vi "Initiaize.vi"(8 "error in (no error)":errorcluster, 11 "Pcal GUI in":refnum<class "Pcal GUI.lvclass">) -> (0 "error out":errorcluster, 3 "Pcal GUI out":refnum<class "Pcal GUI.lvclass">)   [LabVIEW 2015, in "Pcal GUI.lvclass"]
uses:
  Pcal GUI.lvclass
  Pcal GUI.lvclass/Pcal GUI.ctl
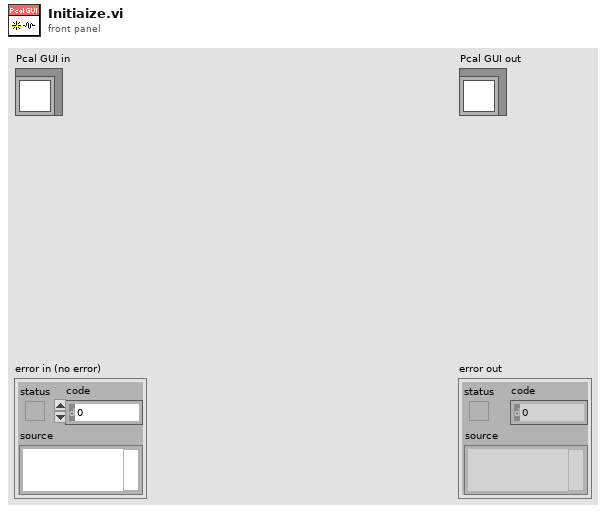
[diagram p1: front panel]
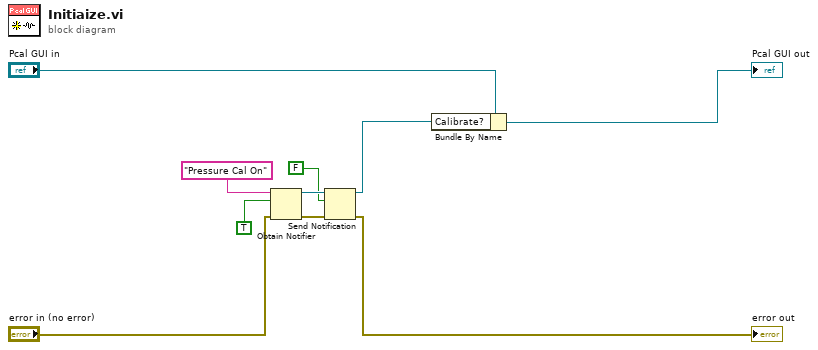
[diagram p0: block diagram]
diagram:
  n1 = Obtain Notifier(name (unnamed)="Pressure Cal On", notification data type=TRUE, error in (no error)="error in (no error)") -> (notifier out=w6:refnum<notifier>, error out=w4:errorcluster)  [unwired: 1 in, 1 out]
  n2 = Send Notification(notification=FALSE, notifier=w6, error in (no error)=w4) -> (notifier out=w3:refnum<notifier>, error out=→"error out":errorcluster)
  n3 = Bundle By Name(cluster="Pcal GUI in", "Calibrate?"=w3) -> (→"Pcal GUI out":refnum<class "Pcal GUI.lvclass">)
